vi "Calculate Error.vi"(10 "X":dbl[](array[numeric]), 11 "Fit Exp in":refnum<class "Fit Exponential.lvclass">) -> (3 "Fit Exp out":refnum<class "Fit Exponential.lvclass">)   [LabVIEW 2012, in "Exponential Fit Library.lvlib" / "Fit Exponential.lvclass"]
doc: "Calculate the error in the fitted coefficient tau according to Halmer et al. [2004, Rev. Sci. Instr.]. The error will be the standard deviation of the fit (with N-3 degrees of freedom) multiplied by the sum of the square of the derivative of the exponential equation at each point in time."
uses:
  Fit Exponential.lvclass
  Fit Exponential.lvclass/Fit Exponential.ctl
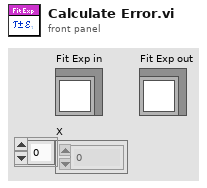
[diagram p1: front panel]
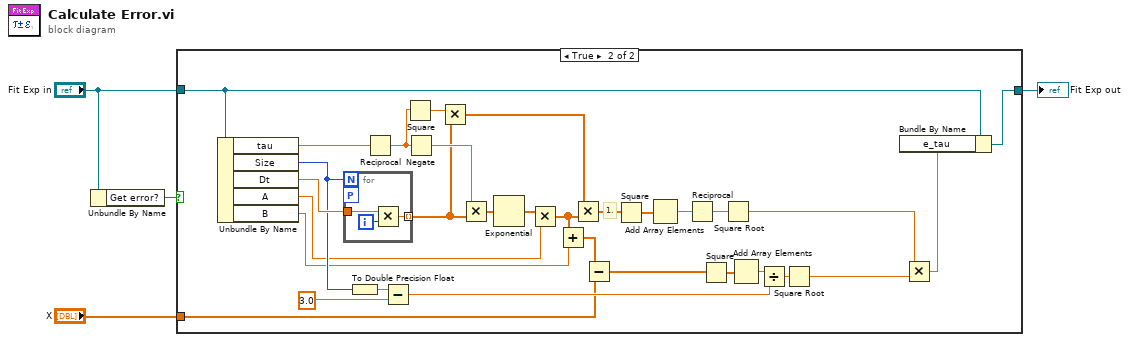
[diagram p0: block diagram]
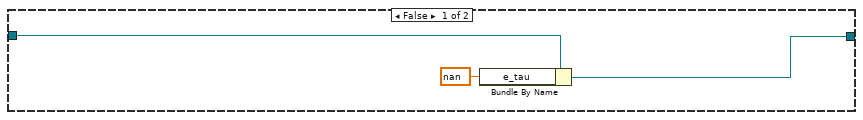
[diagram p2: hidden frame]
diagram:
  n1 = Unbundle By Name("Fit Exp in") -> ("Get error?"=w2:bool)
  n2 = case shown="True" w2 {
    tunnel: [w6 w38] -> w4
    tunnel: "Fit Exp in" -> [w7 w37]
    tunnel: "X" -> [_ w8]
    frame False {
      n3 = Bundle By Name(cluster=w7, "e_tau"=nan ("Output.e_tau")) -> (w6:refnum<class "Fit Exponential.lvclass">)
    }
    frame True {
      # "1."
      n4 = Unbundle By Name(w37) -> ("tau"=w13:dbl, "Size"=w11:i32, "Dt"=w12:dbl, "A"=w10:dbl, "B"=w9:dbl)
      n5 = for {
        N: w11 -> [_]
        tunnel: w12 -> [w40]
        tunnel: [w39] -> w27 mode=indexing
        workers-P: _ -> [_]
        i -> [w41]
        n6 = Multiply(x=w40, y=w41) -> (x*y=w39:dbl)
      }
      n7 = To Double Precision Float(number=w11) -> (double precision float=w35:dbl)
      n8 = Reciprocal(x=w13) -> (1/x=w29:dbl)
      n9 = Subtract(x=w35, y=3.0) -> (x-y=w34:dbl)
      n10 = Square(x=w29) -> (x^2=w28:dbl)
      n11 = Negate(x=w29) -> (-x=w30:dbl)
      n12 = Multiply(x=w28, y=w27) -> (x*y=w26:dbl[])
      n13 = Multiply(x=w30, y=w27) -> (x*y=w31:dbl[])
      n14 = Exponential(1:w31) -> (0:w17:dbl[])
      n15 = Multiply(x=w17, y=w10) -> (x*y=w15:dbl[])
      n16 = Add(x=w15, y=w9) -> (x+y=w16:dbl[])
      n17 = Multiply(x=w26, y=w15) -> (x*y=w25:dbl[])
      n18 = Subtract ("residual")(x=w16, y=w8) -> (x-y=w22:dbl[])
      n19 = Square(x=w25) -> (x^2=w24:dbl[])
      n20 = Add Array Elements(numeric array=w24) -> (sum=w19:dbl)
      n21 = Reciprocal(x=w19) -> (1/x=w18:dbl)
      n22 = Square(x=w22) -> (x^2=w32:dbl[])
      n23 = Square Root(x=w18) -> (sqrt(x)=w23:dbl)
      n24 = Add Array Elements(numeric array=w32) -> (sum=w33:dbl)
      n25 = Divide ("sigma")(x=w33, y=w34) -> (x/y=w21:dbl)
      n26 = Square Root ("sigma")(x=w21) -> (sqrt(x)=w20:dbl)
      n27 = Multiply(x=w23, y=w20) -> (x*y=w14:dbl)
      n28 = Bundle By Name(cluster=w37, "e_tau"=w14) -> (w38:refnum<class "Fit Exponential.lvclass">)
    }
  }
  "Fit Exp out" <- w4
